vi "Set Watchdog Delay.vi"(1 "Delay before PC comms failure closure":u16, 2 "Boolean":bool) -> (0 "result string":string)   [LabVIEW 2009]
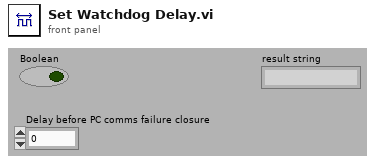
[diagram p1: front panel]
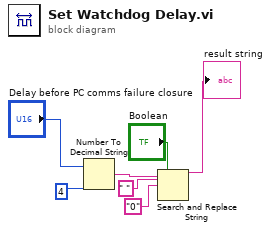
[diagram p0: block diagram]
diagram:
  n1 = Number To Decimal String(number="Delay before PC comms failure closure", width (-)=i16 4) -> (decimal integer string=w7:string)
  n2 = Search and Replace String(replace all?="Boolean", input string=w7, search string=" ", replace string="0") -> (result string=→"result string":string)  [unwired: 4 in, 3 out]
